vi "Initialize Archiving.vi"(8 "error in (no error)":errorcluster, 10 "Timer Handler":T1, 11 "System Configuration":T2) -> (0 "error out":errorcluster, 3 "dup System Configuration":T2)   [LabVIEW 2024]
doc: "Initialize data archiving."
uses:
  Controls/Server/System Configuration.ctl
  Controls/Server/Subsystem Configuration.ctl
  Timer/Timer Handler.ctl
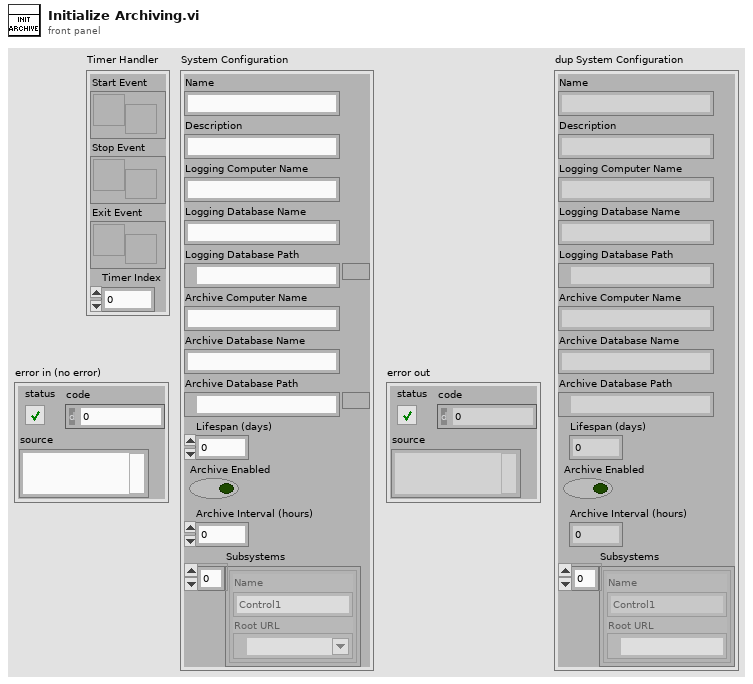
[diagram p1: front panel]
types:
  T1 = typedef "Timer Handler.ctl" = cluster{"Start Event":refnum<user-event>, "Stop Event":refnum<user-event>, "Exit Event":refnum<user-event>, "Timer Index":u32}
  T2 = typedef "System Configuration.ctl" = cluster{"Name":string, "Description":string, "Logging Computer Name":string, "Logging Database Name":string, "Logging Database Path":path, "Archive Computer Name":string, "Archive Database Name":string, "Archive Database Path":path, "Lifespan (days)":u32, "Archive Enabled":bool, "Archive Interval (hours)":u32, "Subsystems":T3[]}
  T3 = typedef "Subsystem Configuration.ctl" = cluster{"Name":string, "Root URL":refnum<k21>}
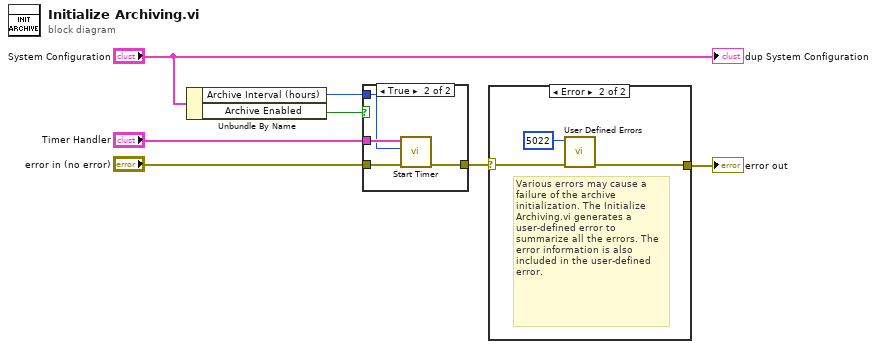
[diagram p0: block diagram]
diagram:
  n1 = Unbundle By Name("System Configuration") -> ("Archive Interval (hours)"=w6:u32, "Archive Enabled"=w5:bool)
  n2 = case shown="True" w5 {
    tunnel: w6 -> [_ w11]
    tunnel: "Timer Handler" -> [_ w12]
    tunnel: [w8 w10] -> w1
    tunnel: "error in (no error)" -> [w8 w9]
    frame False {
    }
    frame True {
      n3 = call "Start Timer.vi"("error in (no error)"=w9, "Timer Interval (hours)"=w11, "Timer Handler"=w12) -> ("error out"=w10:errorcluster)  [unwired: 8 in]
    }
  }
  n4 = case shown="Error" w1 {
    selector: w1 -> [w13 w15]
    tunnel: [w13 w14] -> w2
    frame No Error {
    }
    frame Error {
      # "Various errors may cause a failure of the archive initialization. The Initialize Archiving.vi generates a user-defined error to summarize all the errors. The error information is also included in the user-defined error."
      n5 = call "User Defined Errors.vi"("error in (no error)"=w15, "Error Code (0)"=5022 ("error code (0)")) -> ("error out"=w14:errorcluster)  [unwired: 9 in]
    }
  }
  "error out" <- w2
  "dup System Configuration" <- "System Configuration"
